vi "Solenoid With Compressor.vi"() -> ()   [LabVIEW 2013]
doc: "Solenoid With Compressor Example \n\nThis example willl start monitoring the pressure of the system which starts the compressor if a fall in pressure is registered."
uses:
  <vilib>/Rock Robotics/WPI/Solenoid/WPI_SolenoidChannel.ctl
  <vilib>/Rock Robotics/SystemInterfaces/DIO/FPGA_DIOChannel.ctl
  <vilib>/Rock Robotics/SystemInterfaces/DIO/FPGA_DIORelayChannel.ctl
  <vilib>/Rock Robotics/SystemInterfaces/Typedef/FPGA_TypedefDigitalModule.ctl
  <vilib>/Rock Robotics/WPI/Solenoid/WPI_SolenoidValue.ctl
  <vilib>/Rock Robotics/WPI/Solenoid/WPI_SolenoidOpenSingle.vi
  <vilib>/Rock Robotics/WPI/Solenoid/WPI_SolenoidSetEnum.vi
panel:
  in  "Pressure Switch\nand Relay Module":T1
  in  "Relay Channel":T2
  in  "Pressure Switch Channel":T3
  in  "Solenoid Channel":T4
  out "Compressor Monitoring?":bool
  in  "stop":bool
  in  "Solenoid":bool
  # "Set these inputs before running."
  # "This can be set while running."
  # "Output information"
  # "Wiring Diagram for Digital Sidecar connected to an NI 9403"
  # "(-)"
  # "B"
  # "A"
  # "8\n7\n6\n5\n4\n3\n2\n1"
  # "Pressure\nSwitch"
  # "RELAY"
  # "Connect\nPower\nHere"
  # "Connect\nCompressor\nHere"
  # "GND"
  # "M-"
  # "SPIKE"
  # "12V"
  # "M+"
  # "B"
  # "20A"
  # "fuse"
  # "PWM cable"
  # "NC"
  # "C"
  # "PWR"
  # "SIG"
  # "(-)"
  # "14\n13\n12\n11\n10\n9\n8\n7\n6\n5\n4\n3\n2\n1"
  # "DIGITAL I/O"
  # "Digital Sidecar"
  # "Wiring Diagram for Solenoid Breakout connected to an NI 9472"
  # "GND"
  # "SIG"
  # "8\n7\n6\n5\n4\n3\n2\n1"
  # "Solenoid"
  # "Solenoid\nGround"
  # "+"
  # "12V from\nbattery"
  # "-"
  # "\"power good\"\n  LED"
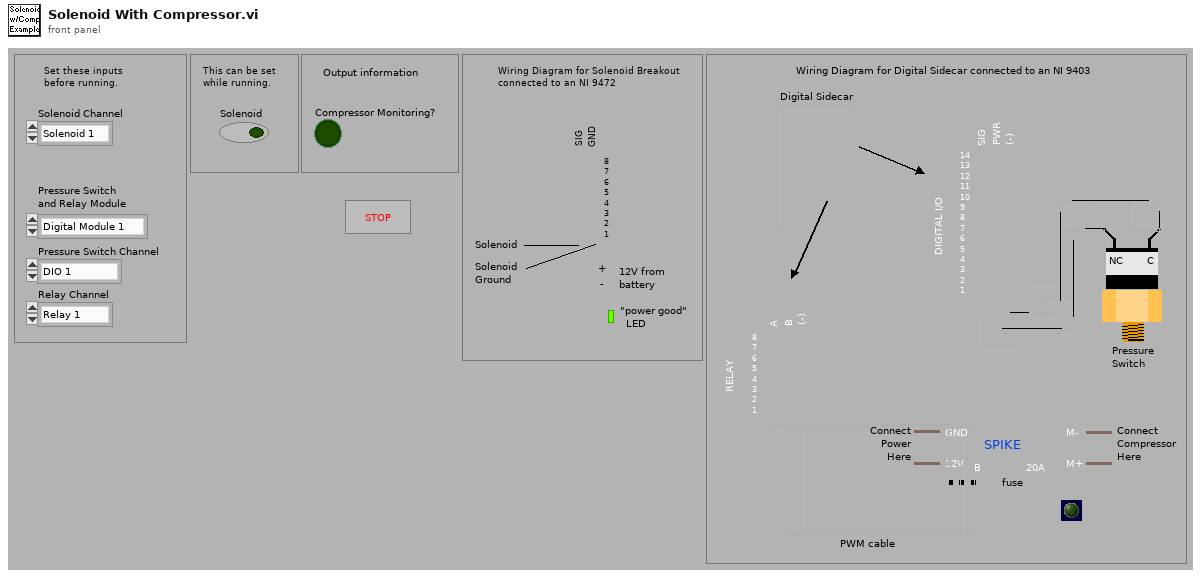
[diagram p1: front panel]
types:
  T1 = typedef "FPGA_TypedefDigitalModule.ctl" = enum16{"Digital Module 1", "Digital Module 2"}
  T2 = typedef "FPGA_DIORelayChannel.ctl" = enum8{"Relay 1", "Relay 2", "Relay 3", "Relay 4", "Relay 5", "Relay 6", "Relay 7", "Relay 8", "Invalid"}
  T3 = typedef "FPGA_DIOChannel.ctl" = enum8{"DIO 1", "DIO 2", "DIO 3", "DIO 4", "DIO 5", "DIO 6", "DIO 7", "DIO 8", "DIO 9", "DIO 10", "DIO 11", "DIO 12", "DIO 13", "DIO 14", "Invalid"}
  T4 = typedef "WPI_SolenoidChannel.ctl" = enum8{"Solenoid 1", "Solenoid 2", "Solenoid 3", "Solenoid 4", "Solenoid 5", "Solenoid 6", "Solenoid 7", "Solenoid 8", "Invalid"}
  T5 = typedef "WPI_CompressorDevRef.ctl" = cluster{"DevStatus":errorcluster, "DigitalInputDevRef":T6, "RelayDevRef":T7}
  T6 = typedef "WPI_DigitalInputDevRef.ctl" = cluster{"DevStatus":errorcluster, "DIO Channel":T3, "Digital Module":T1}
  T7 = typedef "WPI_RelayDevRef.ctl" = cluster{"DevStatus":errorcluster, "Relay Channel":T2, "Digital Module":T1, "Relay Direction":T8}
  T8 = typedef "WPI_RelayDirection.ctl" = enum16{"Both directions", "Forward only", "Reverse only"}
  T9 = typedef "WPI_SolenoidDevRef.ctl" = cluster{"DevStatus":errorcluster, "Solenoid Module":T10, "Forward Solenoid Channel":T4, "Reverse Solenoid Channel":T4}
  T10 = typedef "FPGA_TypedefSolenoidModule.ctl" = enum16{"Solenoid Module 1", "Solenoid Module 2"}
  T11 = typedef "WPI_SolenoidValue.ctl" = enum16{"Off", "On", "Forward", "Reverse"}
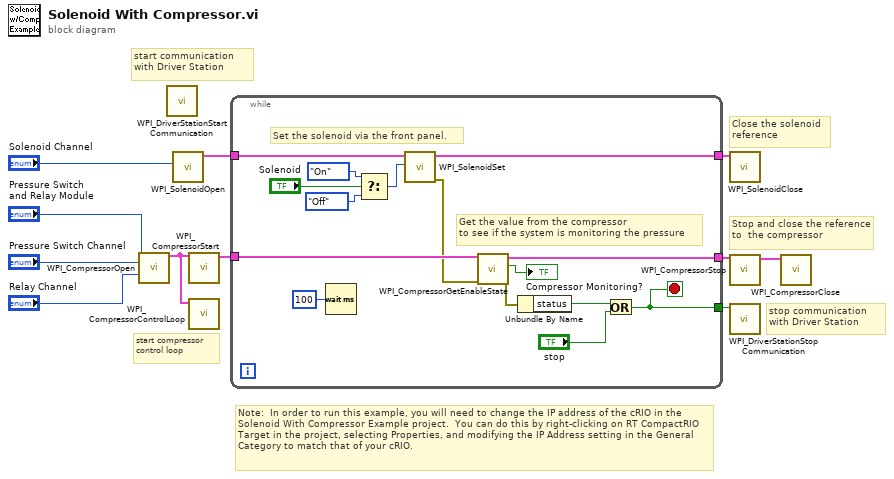
[diagram p0: block diagram]
diagram:
  # "start compressor control loop"
  # "stop communication with Driver Station"
  # "start communication with Driver Station"
  # "Note:  In order to run this example, you will need to change the IP address of the cRIO in the Solenoid With Compressor Example project.  You can do this by right-clicking on RT CompactRIO Target in the project, selecting Properties, and modifying the IP Address setting in the General Category to match that of your cRIO."
  # "Close the solenoid\nreference"
  # "Stop and close the reference to  the compressor"
  n1 = call <vilib>:"WPI_CompressorOpen.vi"("Pressure Switch Digital Module (Module 1)"="Pressure Switch\nand Relay Module", "Pressure Switch DIO Channel"="Pressure Switch Channel", "Relay Channel"="Relay Channel") -> ("CompressorDevRef"=w1:T5)  [unwired: 2 in, 10 out]
  n2 = call <vilib>:"WPI_DriverStationStart Communication.vi"() -> ()  [unwired: 1 in, 11 out]
  n3 = call-poly <vilib>:"WPI_SolenoidOpen.vi"("Solenoid Channel"="Solenoid Channel") -> ("SolenoidDevRef"=w10:T9)  [unwired: 2 in, 8 out]
  n4 = call <vilib>:"WPI_CompressorStart.vi"("CompressorDevRef"=w1) -> ("CompressorDevRef"=w7:T5)  [unwired: 1 in, 9 out]
  n5 = call <vilib>:"WPI_CompressorControlLoop.vi"("CompressorDevRef"=w1) -> ()  [unwired: 11 in]
  n6 = while {
    tunnel: w10 -> [w26]
    tunnel: [w22] -> w9
    tunnel: w7 -> [w25]
    tunnel: [w24] -> w6
    tunnel: [w20] -> w3
    stop <- w20 stop-if-true
    # "Get the value from the compressor \nto see if the system is monitoring the pressure"
    # "Set the solenoid via the front panel."
    n7 = Wait (ms)(milliseconds to wait=u32 100) -> ()  [unwired: 1 out]
    n8 = Select(t=WPI_SolenoidValue."On" ("Value"), s="Solenoid", f=WPI_SolenoidValue."Off" ("Value")) -> (s? t:f=w12:T11)
    n9 = call-poly <vilib>:"WPI_SolenoidSet.vi"("Value"=w12, "SolenoidDevRef"=w26) -> ("error out"=w21:errorcluster, "SolenoidDevRef"=w22:T9)  [unwired: 1 in, 7 out]
    n10 = call <vilib>:"WPI_CompressorGetEnableState.vi"("error in (no error)"=w21, "CompressorDevRef"=w25) -> ("error out"=w18:errorcluster, "Enabled"=→"Compressor Monitoring?":bool, "CompressorDevRef"=w24:T5)  [unwired: 7 out]
    n11 = Unbundle By Name(w18) -> ("status"=w17:bool)
    n12 = Or(x=w17, y="stop") -> (x .or. y?=w20:bool)
  }
  n13 = call <vilib>:"WPI_SolenoidClose.vi"("SolenoidDevRef"=w9) -> ()  [unwired: 1 in, 10 out]
  n14 = call <vilib>:"WPI_CompressorStop.vi"("CompressorDevRef"=w6) -> ("CompressorDevRef"=w8:T5)  [unwired: 1 in, 9 out]
  n15 = call <vilib>:"WPI_DriverStationStop Communication.vi"("StopCommunication"=w3) -> ()  [unwired: 1 in, 10 out]
  n16 = call <vilib>:"WPI_CompressorClose.vi"("CompressorDevRef"=w8) -> ()  [unwired: 1 in, 10 out]
